vi "WILT Populate Status Control.vi"(9 "Index":i32, 10 "GUI Aisle 1 (SLAT) in":T1[](array[typedef]) {"Night Cycle Count" format="%04d"; "Day Cycle Count" format="%04d"}, 11 "Raw Data From File":string[](array[string])) -> (3 "GUI Aisle 1 (SLAT) out":T1[](array[typedef]) {"Night Cycle Count" format="%04d"; "Day Cycle Count" format="%04d"})   [LabVIEW 2016]
uses:
  Type Definitions/WILT Dryer.ctl
  Type Definitions/WILT Dryer Details.ctl
  Type Definitions/WILT Agilent Channel Definition.ctl
  Type Definitions/WILT DAQ Data.ctl
panel:
  # "Day"
  # "Night"
  # "Day"
  # "Night"
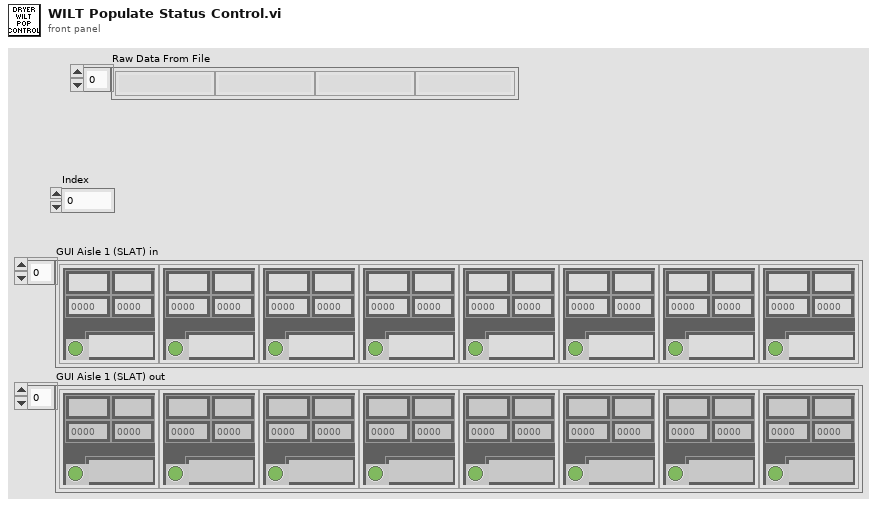
[diagram p1: front panel]
types:
  T1 = typedef "WILT Dryer.ctl" = cluster{"Lab ID":string, "Day Cycle Count":i32, "Station Label":string, "Dryer Details":T2, "Status Color":u32, "Invisible Button":bool, "Night Cycle Count":i32, "Station Index":i32, "Cycle Index":string, "Audit Alert":bool, "Agilent Channel Definition":T3, "DAQ Data":T4}
  T2 = typedef "WILT Dryer Details.ctl" = cluster{"Station":string, "Lab ID":string, "TR Number":string}
  T3 = typedef "WILT Agilent Channel Definition.ctl" = cluster{"Channel":string, "Station":string, "Label":string, "Agilent Station":string, "Data":dbl}
  T4 = typedef "WILT DAQ Data.ctl" = cluster{"L1 Current":dbl, "L2 Current":dbl, "Temperature  Deg F (TC)":dbl, "Volts":dbl, "Volts (208)":dbl, "SW (208)":dbl}
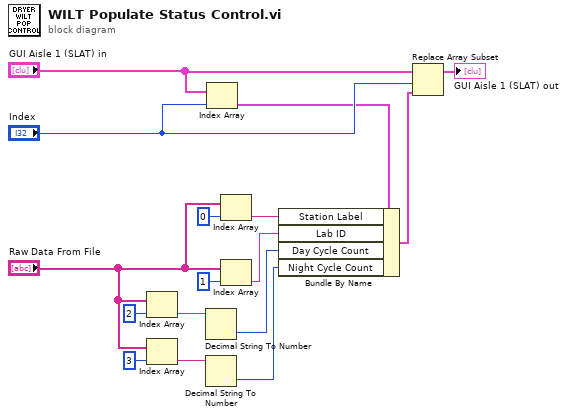
[diagram p0: block diagram]
diagram:
  n1 = Index Array(array="Raw Data From File", index=2) -> (element=w9:string)
  n2 = Index Array(array="Raw Data From File", index=3) -> (element=w11:string)
  n3 = Decimal String To Number(string=w9) -> (number=w10:i32)  [unwired: 2 in, 1 out]
  n4 = Decimal String To Number(string=w11) -> (number=w12:i32)  [unwired: 2 in, 1 out]
  n5 = Index Array(array="GUI Aisle 1 (SLAT) in", index="Index") -> (element=w1:T1)
  n6 = Index Array(array="Raw Data From File", index=0) -> (element=w7:string)
  n7 = Index Array(array="Raw Data From File", index=1) -> (element=w8:string)
  n8 = Bundle By Name(cluster=w1, "Station Label"=w7, "Lab ID"=w8, "Day Cycle Count"=w10, "Night Cycle Count"=w12) -> (w13:T1)
  n9 = Replace Array Subset(array="GUI Aisle 1 (SLAT) in", new element=w13, index="Index") -> (→"GUI Aisle 1 (SLAT) out":T1[])
